vi "Test CycloneDX BOM from Source.vi"() -> ()   [LabVIEW 2017]
uses:
  CycloneDX/CycloneDX SBOM/CycloneDX SBOM.lvclass
  C:/LabVIEW Working Directory/labview-cyclonedx-sbom/Source/CycloneDX/CycloneDX JSON/CycloneDX JSON.lvclass
  CycloneDX/CycloneDX JSON/CycloneDX Types.ctl
  CycloneDX/CycloneDX Component/CycloneDX Component.lvclass
  CycloneDX/CycloneDX JSON/CycloneDX JSON.lvclass
  LabVIEW Installer Support/LabVIEW Installer Support.lvlib
  VIP Support/VIP SBOM Support.lvlib
  <vilib>/JDP Science/JSONtext/JSONtext.lvlib
panel:
  in  "Installer Build Specification Name":string caption="Installer Build Specification Name (\"\" = use first installer in project)"
  in  "VI Packages - VIPC or Project Path":path
  in  "LabVIEW Project Path":path caption="LabVIEW Project Path (for additional installer scanning)"
  out "CycloneDX SBOM out":refnum<class "CycloneDX SBOM.lvclass">
  out "error out":errorcluster
  out "JSON":string
  # "Example CycloneDX SBOM Generation using constant(s) for dependencies"
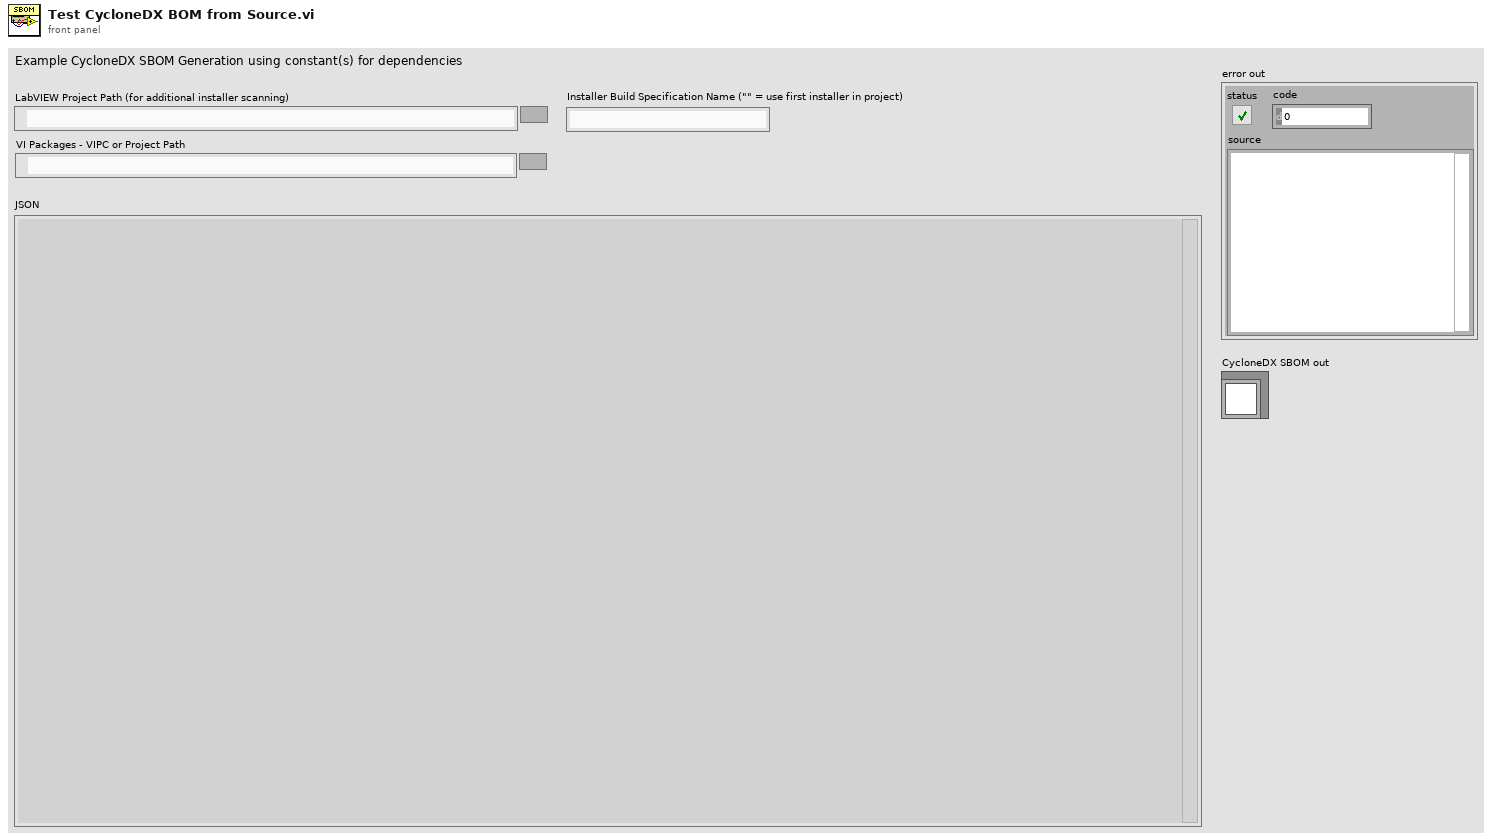
[diagram p1: front panel]
types:
  T1 = typedef "LabVIEW CycloneDX SBOM.lvlib/CycloneDX JSON.lvclass/CycloneDX Types.ctl" = enum16{"application", "framework", "library", "container", "platform", "operating-system", "device", "device-driver", "firmware", "file", "machine-learning-model", "data"}
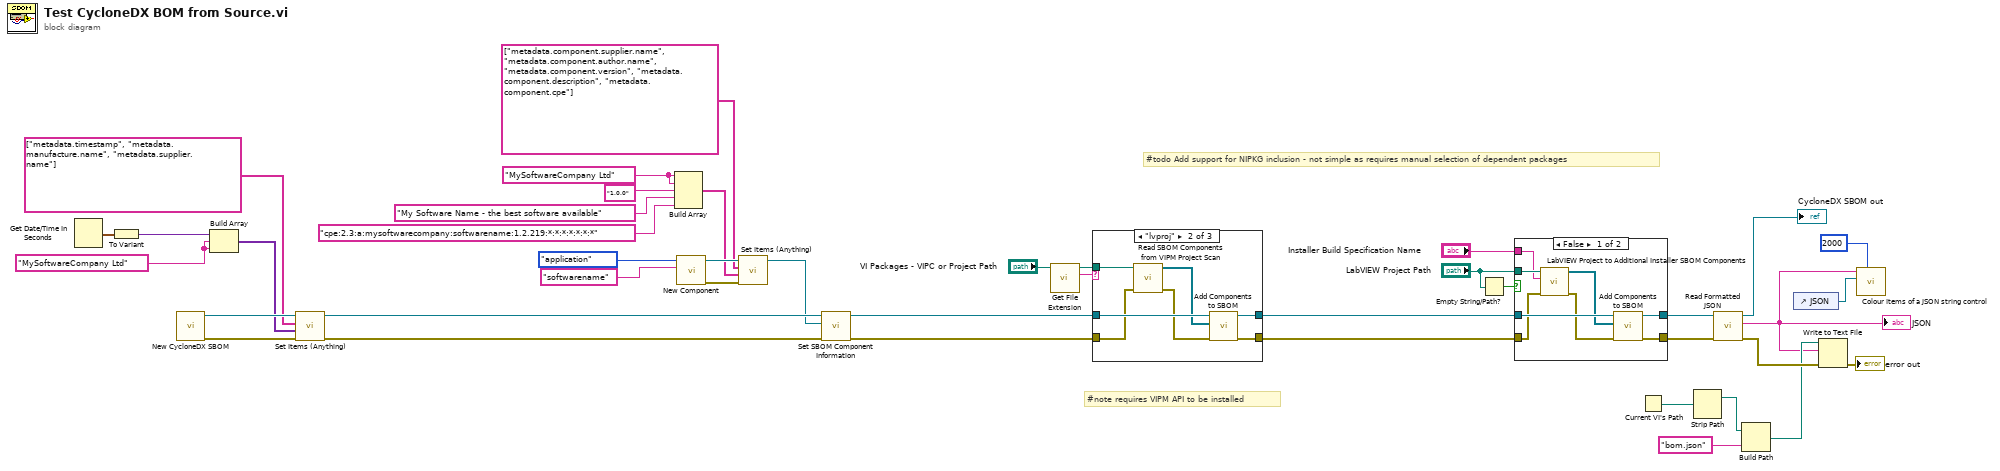
[diagram p0: block diagram]
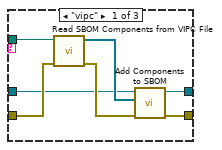
[diagram p2: hidden frame]
diagram:
  w14 = "MySoftwareCompany Ltd"
  w22 = "MySoftwareCompany Ltd"
  # "#note requires VIPM API to be installed"
  # "#todo Add support for NIPKG inclusion - not simple as requires manual selection of dependent packages"
  n1 = Get Date/Time In Seconds() -> (seconds since 1Jan1904=w25:timestamp)
  n2 = To Variant(anything=w25) -> (Variant=w24:variant)
  n3 = call "New CycloneDX SBOM.vi"() -> ("error out"=w28:errorcluster, "CycloneDX SBOM out"=w27:refnum<class "CycloneDX SBOM.lvclass">)  [unwired: 10 in]
  n4 = Build Array(w24, w22, w22) -> (w23:variant[])
  n5 = call "Set Items (Anything).vi"("error in (no error)"=w28, "Value"=w23, "Item Paths"=string[] ["metadata.timestamp", "metadata.manufacture.name", "metadata.supplier.name"] ("Object (or Item) Path"), "CycloneDX SBOM in"=w27) -> ("error out"=w20:errorcluster, "CycloneDX SBOM out"=w21:refnum<class "CycloneDX SBOM.lvclass">)  [unwired: 6 in]
  n6 = Build Array(w14, w14, "1.0.0", "My Software Name - the best software available", "cpe:2.3:a:mysoftwarecompany:softwarename:1.2.219:*:*:*:*:*:*:*") -> (w10:string[])
  n7 = call "New Component.vi"("name"="softwarename", "type"=CycloneDX_Types."application") -> ("error out"=w17:errorcluster, "CycloneDX Component out"=w16:refnum<class "CycloneDX Component.lvclass">)  [unwired: 8 in]
  n8 = call "Set Items (Anything).vi"("error in (no error)"=w17, "Value"=w10, "Item Paths"=string[] ["metadata.component.supplier.name", "metadata.component.author.name", "metadata.component.version", "metadata.component.description", "metadata.component.cpe"] ("Object (or Item) Path"), "CycloneDX SBOM in"=w16) -> ("CycloneDX SBOM out"=w7:refnum<class "CycloneDX Component.lvclass">)  [unwired: 6 in, 1 out]
  n9 = call "Set SBOM Component Information.vi"("error in (no error)"=w20, "CycloneDX Component"=w7, "CycloneDX SBOM in"=w21) -> ("error out"=w9:errorcluster, "CycloneDX SBOM out"=w8:refnum<class "CycloneDX SBOM.lvclass">)  [unwired: 7 in]
  n10 = call <vilib>:"Get File Extension.vi"("file"="VI Packages - VIPC or Project Path") -> ("lowercase file extension"=w1:string, "dup file"=w2:path)  [unwired: 6 in, 3 out]
  n11 = case shown="\"lvproj\"" w1 {
    tunnel: [w49 w56 w57] -> w36
    tunnel: [w46 w55 w58] -> w33
    tunnel: w9 -> [w45 w53 w58]
    tunnel: w8 -> [w44 w54 w57]
    tunnel: w2 -> [w43 w52 _]
    frame "vipc" {
      n12 = call "Read SBOM Components from VIPC File.vi"("error in (no error)"=w45, "VIPC path"=w43) -> ("error out"=w48:errorcluster, "SBOM Components out"=w47:refnum<class "CycloneDX Component.lvclass">[])  [unwired: 8 in]
      n13 = call "Add Components to SBOM.vi"("error in (no error)"=w48, "Component(s) to add"=w47, "CycloneDX SBOM in"=w44) -> ("error out"=w46:errorcluster, "CycloneDX SBOM out"=w49:refnum<class "CycloneDX SBOM.lvclass">)  [unwired: 7 in]
    }
    frame "lvproj" {
      n14 = call "Read SBOM Components from VIPM Project Scan.vi"("error in (no error)"=w53, "LabVIEW project path"=w52) -> ("error out"=w51:errorcluster, "SBOM Components out"=w50:refnum<class "CycloneDX Component.lvclass">[])  [unwired: 8 in]
      n15 = call "Add Components to SBOM.vi"("error in (no error)"=w51, "Component(s) to add"=w50, "CycloneDX SBOM in"=w54) -> ("error out"=w55:errorcluster, "CycloneDX SBOM out"=w56:refnum<class "CycloneDX SBOM.lvclass">)  [unwired: 7 in]
    }
    frame Default {
    }
  }
  n16 = Empty String/Path?(string/path="LabVIEW Project Path") -> (empty?=w5:bool)
  n17 = case shown="False" w5 {
    tunnel: w36 -> [w66 w67]
    tunnel: [w65 w68] -> w35
    tunnel: [w64 w67] -> w34
    tunnel: w33 -> [w63 w68]
    tunnel: "LabVIEW Project Path" -> [w60 _]
    tunnel: "Installer Build Specification Name" -> [w59 _]
    frame False {
      n18 = call "LabVIEW Project to Additional Installer SBOM Components.vi"("error in (no error)"=w63, "Build Specification Name (\"\" = first installer)"=w59, "LabVIEW Project Path"=w60) -> ("error out"=w62:errorcluster, "Installer components"=w61:refnum<class "CycloneDX Component.lvclass">[])  [unwired: 7 in]
      n19 = call "Add Components to SBOM.vi"("error in (no error)"=w62, "Component(s) to add"=w61, "CycloneDX SBOM in"=w66) -> ("error out"=w65:errorcluster, "CycloneDX SBOM out"=w64:refnum<class "CycloneDX SBOM.lvclass">)  [unwired: 7 in]
    }
    frame True {
    }
  }
  n20 = Current VI's Path() -> (path=w41:path)
  n21 = Strip Path(path=w41) -> (stripped path=w40:path)  [unwired: 1 out]
  n22 = call "Read Formatted JSON.vi"("error in (no error)"=w35, "CycloneDX SBOM in"=w34) -> ("error out"=w42:errorcluster, "JSON"=w32:string, "CycloneDX SBOM out"=→"CycloneDX SBOM out":refnum<class "CycloneDX SBOM.lvclass">)  [unwired: 7 in]
  "JSON" <- w32
  n23 = Build Path(base path=w40, name or relative path="bom.json") -> (appended path=w38:path)
  n24 = control-ref of="JSON"() -> (w30:refnum<vi>)
  n25 = Write to Text File(file (use dialog)=w38, text=w32, error in=w42) -> (error out=→"error out":errorcluster)  [unwired: 1 in, 2 out]
  n26 = call <vilib>:"Colour Items of a JSON string control.vi"("Maximum UI Property calls"=2000, "String Control"=w30, "JSON"=w32) -> ()  [unwired: 9 in]
